vi "CS_cRIO-PB_DP-Master_StartStop.vi"(0 "FPGA VI Reference":T2, 5 "DP-Master":enum16{"Start", "Stop"}(ring), 11 "Error":errorcluster) -> (4 "FPGA VI Reference out":T2, 8 "Slave Info List":T1(array[cluster]), 15 "Error out":errorcluster)   [LabVIEW 2013, in "dynamic profibus.lvlib"]
doc: "Starts/Stops the cRIO-PB as Profibus Master.\n\nFPGA VI Reference:\nReference of the FPGA VI.\n\nDP-Master:\nThe \"Start\" mode activates the cRIO-PB as DP-Master Class 1 and Class 2.\nThe \"Stop\" mode resets the cRIO-PB.\n\nSlave Info List:\nThe list contains additional information about input and output lengths of the configured DP-Slaves.\n\nFPGA VI Reference out:\nIs a copy of the FPGA VI Reference .\n\nError in:\nPreceding error conditions. If an error has already occurred, the VI returns the value of the error in Error out.\n\nError out:\nError: TRUE if an error occurred.\nStatus: Error code\nInfo: Error description"
uses:
  dynamic profibus.lvlib
  CS_cRIO-PB_DP-Master_FPGA-Reference.ctl
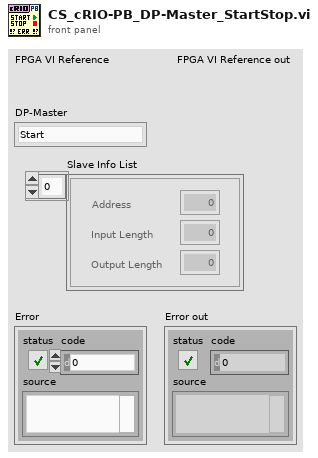
[diagram p1: front panel]
types:
  T1 = cluster{"Address":i8, "Input Length":u8, "Output Length":u8}[]
  T2 = typedef "dynamic profibus.lvlib/CS_cRIO-PB_DP-Master_FPGA-Reference.ctl" = refnum<k20>
  T3 = enum16{"Start/Stop DP-Master", "Get Input Data", "Set Output Data", "Get Output Data", "Get Diagnostic Data", "Read/Write Data", "Read Diagnostic Data", "Get DPV1 Data", "Set DPV1 Data", "Read/Write DPV1 Data"}
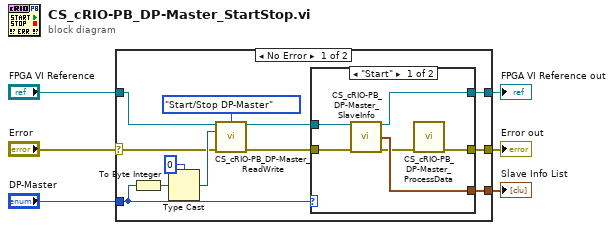
[diagram p0: block diagram]
diagram:
  n1 = case shown="No Error" "Error" {
    selector: "Error" -> [w13 w27]
    tunnel: "FPGA VI Reference" -> [w10 w28]
    tunnel: [w15 w27] -> w5
    tunnel: [w16 w28] -> w4
    tunnel: "DP-Master" -> [w18 _]
    tunnel: [w14 _] -> w1
    frame No Error {
      n2 = To Byte Integer(number=w18) -> (8bit integer=w7:i8)
      n3 = Type Cast(type=i8 0, x=w7) -> (*(type *) &x=w17:i8)
      n4 = call "CS_cRIO-PB_DP-Master_ReadWrite.vi"("FPGA VI Reference"=w10, "Mode"=T3."Start/Stop DP-Master", "Slave"=w17, "Error"=w13) -> ("FPGA VI Reference out"=w9:T2, "Error out"=w12:errorcluster)  [unwired: 8 in, 2 out]
      n5 = case shown="\"Start\"" w18 {
        tunnel: w12 -> [w23 w25]
        tunnel: w9 -> [w22 w26]
        tunnel: [w21 w26] -> w16
        tunnel: [w19 w25] -> w15
        tunnel: [w24 _] -> w14
        frame "Start" {
          n6 = call "CS_cRIO-PB_DP-Master_SlaveInfo.vi"("FPGA VI Reference"=w22, "Error"=w23) -> ("FPGA VI Reference out"=w21:T2, "Slave Info List"=w24:T1, "Error out"=w20:errorcluster)  [unwired: 11 in]
          n7 = call "CS_cRIO-PB_DP-Master_ProcessData.vi"("Error"=w20) -> ("Error out"=w19:errorcluster)  [unwired: 12 in, 2 out]
        }
        frame "Stop" {
        }
      }
    }
    frame Error {
    }
  }
  "Error out" <- w5
  "FPGA VI Reference out" <- w4
  "Slave Info List" <- w1
